vi "Force.vi"() -> ()   [LabVIEW 2017]
panel:
  out "Feedback_ON_OFF":bool
  out "Fy":dbl
  out "Fx":dbl
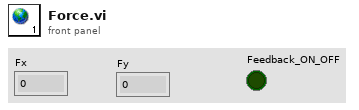
[diagram p1: front panel]
diagram:
